vi "Power Output Compare and Coerce Stimulus.vi"(6 "Driver Ref (null)":T1, 8 "error in (no error)":errorcluster, 10 "Flat TestSetDef Params":string, 11 "PV Test Parameters":T2={"Stimulus"={"Frequency Type"=enum."Band Edges", "Frequency Ranges"=[], "TX 1 Frequency (MHz)"={"Min"=0.0, "Max"=0.0}, "TX 2 Frequency (MHz)"={"Min"=0.0, "Max"=0.0}, "RX Frequency (MHz)"={"Min"=0.0, "Max"=0.0}, "Pad Model Number"="", "Pad Serial Number"="", "Pad Values"=[]}, "Measurement"={"DUT Port"=enum."Port 1", "Direction"=0, "Frequency Step Size"=0}, "Display"={"Frequency"={"Min"=-1.0, "Max"=-1.0}, "Power"={"Min"=-1, "Max"=-1}}, "Limit"={"Min Power (dBm)"=44.0}, "Calibration"={"Calibrated?"=FALSE}} {"Measurement"."Frequency Step Size" items=["0.2", "0.4", "1.0", "2.0", "4.0"]; "Measurement"."Direction" items=["Reverse", "Forward", "Auxiliary"]}) -> (0 "error out":errorcluster, 3 "Corrected Test Params":T2={"Stimulus"={"Frequency Type"=enum."Band Edges", "Frequency Ranges"=[], "TX 1 Frequency (MHz)"={"Min"=0.0, "Max"=0.0}, "TX 2 Frequency (MHz)"={"Min"=0.0, "Max"=0.0}, "RX Frequency (MHz)"={"Min"=0.0, "Max"=0.0}, "Pad Model Number"="", "Pad Serial Number"="", "Pad Values"=[]}, "Measurement"={"DUT Port"=enum."Port 1", "Direction"=0, "Frequency Step Size"=0}, "Display"={"Frequency"={"Min"=-1.0, "Max"=-1.0}, "Power"={"Min"=-1, "Max"=-1}}, "Limit"={"Min Power (dBm)"=44.0}, "Calibration"={"Calibrated?"=FALSE}} {"Measurement"."Frequency Step Size" items=["0.2", "0.4", "1.0", "2.0", "4.0"]; "Measurement"."Direction" items=["Reverse", "Forward", "Auxiliary"]}, 4 "TestSetDef":T11={"General"={"ID"=0, "Model"="", "Dual Port?"=FALSE, "Options"="", "Options"={"E"=FALSE, "K"=FALSE, "H"=FALSE, "W"=FALSE, "F"=FALSE}, "Cal File"=path ""}, "Receiver"={"Fstart, MHz"=0.0, "Fstop MHz"=0.0, "Fstep MHz"=0.0, "IF, MHz"=0.0}, "RX Band"={"Fstart, MHz"=0.0, "Fstop MHz"=0.0}, "TX 1"={"Fstart, MHz"=0.0, "Fstop MHz"=0.0, "Pmax, dBm"=0.0, "Pstep, dB"=0.0}, "TX 2"={"Fstart, MHz"=0.0, "Fstop MHz"=0.0, "Pmax, dBm"=0.0, "Pstep, dB"=0.0}, "Low-side?"=TRUE})   [LabVIEW 2011]
uses:
  SI.LIB/PIM.LIB/HW IO/Test Set Definition.ctl
  TypeDefs/Power Output Test Parameters.ctl
  TypeDefs/Power Output Stimulus Parameters.ctl
  TypeDefs/Power Output Measurement Parameters.ctl
  SI.LIB/PIM.LIB/HW IO/DUTport.ctl
  SI.LIB/PIM.LIB/HW IO/MeasMode.ctl
  SI.LIB/PIM.LIB/HW IO/PIM Sweep Step Size.ctl
  TypeDefs/Power Output Display Parameters.ctl
  TypeDefs/Power Output Limit Parameters.ctl
  TypeDefs/Power Output Calibration State.ctl
  drivers/PIM/PIM Driver Ref.ctl
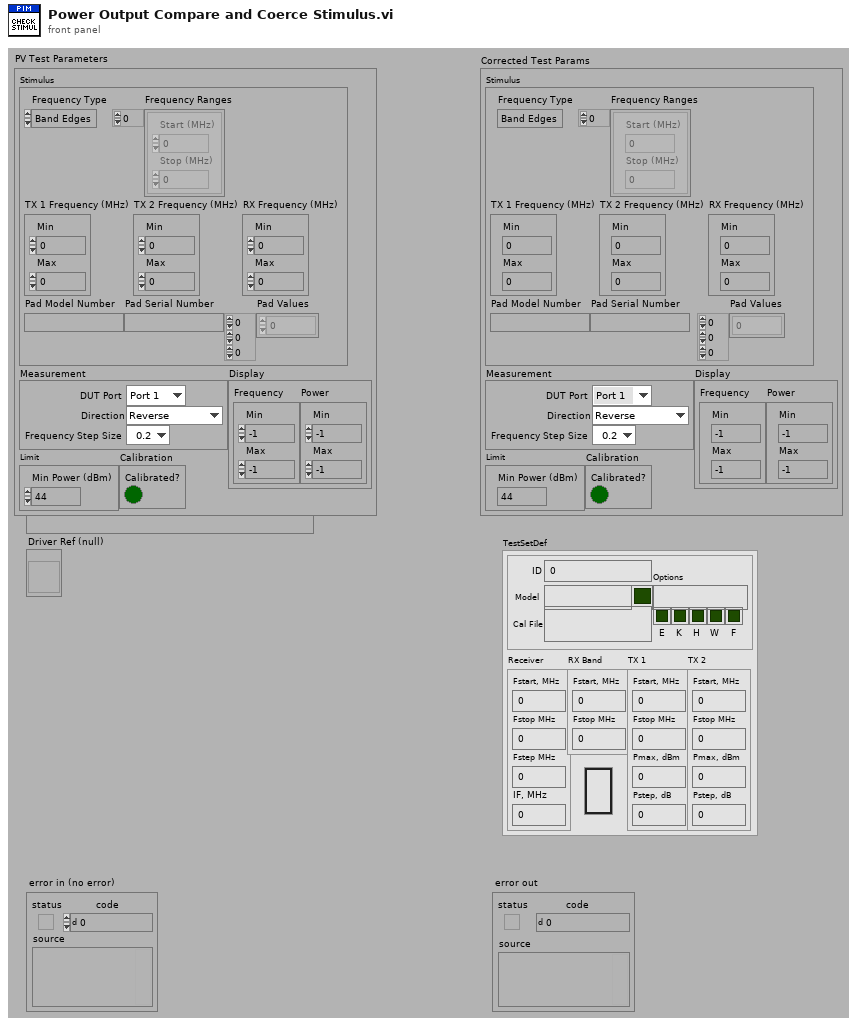
[diagram p1: front panel]
types:
  T1 = typedef "PIM Driver Ref.ctl" = refnum<vi>
  T2 = typedef "Power Output Test Parameters.ctl" = cluster{"Stimulus":T3, "Measurement":T4, "Display":T8, "Limit":T9, "Calibration":T10}
  T3 = typedef "Power Output Stimulus Parameters.ctl" = cluster{"Frequency Type":enum16{"Band Edges", "Custom"}, "Frequency Ranges":cluster{"Start (MHz)":dbl, "Stop (MHz)":dbl}[], "TX 1 Frequency (MHz)":cluster{"Min":dbl, "Max":dbl}, "TX 2 Frequency (MHz)":cluster{"Min":dbl, "Max":dbl}, "RX Frequency (MHz)":cluster{"Min":dbl, "Max":dbl}, "Pad Model Number":string, "Pad Serial Number":string, "Pad Values":dbl[][][]}
  T4 = typedef "Power Output Measurement Parameters.ctl" = cluster{"DUT Port":T5, "Direction":T6, "Frequency Step Size":T7}
  T5 = typedef "DUTport.ctl" = enum16{"Port 1", "Port 2"}
  T6 = typedef "MeasMode.ctl" = u16
  T7 = typedef "PIM Sweep Step Size.ctl" = u16
  T8 = typedef "Power Output Display Parameters.ctl" = cluster{"Frequency":cluster{"Min":dbl, "Max":dbl}, "Power":cluster{"Min":i32, "Max":i32}}
  T9 = typedef "Power Output Limit Parameters.ctl" = cluster{"Min Power (dBm)":dbl}
  T10 = typedef "Power Output Calibration State.ctl" = cluster{"Calibrated?":bool}
  T11 = typedef "Test Set Definition.ctl" = cluster{"General":cluster{"ID":u32, "Model":string, "Dual Port?":bool, "Options":string, "Options":cluster{"E":bool, "K":bool, "H":bool, "W":bool, "F":bool}, "Cal File":path}, "Receiver":cluster{"Fstart, MHz":dbl, "Fstop MHz":dbl, "Fstep MHz":dbl, "IF, MHz":dbl}, "RX Band":cluster{"Fstart, MHz":dbl, "Fstop MHz":dbl}, "TX 1":cluster{"Fstart, MHz":dbl, "Fstop MHz":dbl, "Pmax, dBm":dbl, "Pstep, dB":dbl}, "TX 2":cluster{"Fstart, MHz":dbl, "Fstop MHz":dbl, "Pmax, dBm":dbl, "Pstep, dB":dbl}, "Low-side?":bool}
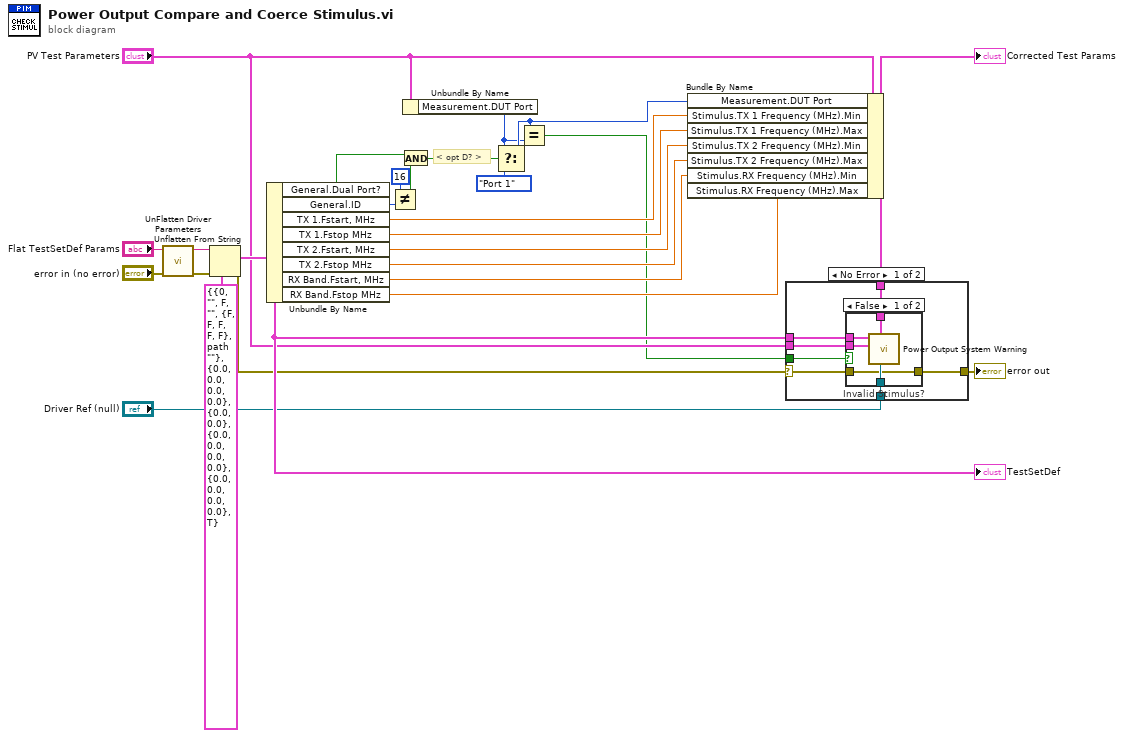
[diagram p0: block diagram]
diagram:
  # "< opt D? >"
  n1 = call "UnFlatten Driver Parameters.vi"("error in (no error)"="error in (no error)", "Flattened Driver Parameters with Version (\"\")"="Flat TestSetDef Params") -> ("error out"=w22:errorcluster, "Flat Driver Parameters"=w24:string)  [unwired: 4 out]
  n2 = Unflatten From String(type=T11 {"General"={"ID"=0, "Model"="", "Dual Port?"=FALSE, "Options"="", "Options"={"E"=FALSE, "K"=FALSE, "H"=FALSE, "W"=FALSE, "F"=FALSE}, "Cal File"=path ""}, "Receiver"={"Fstart, MHz"=0.0, "Fstop MHz"=0.0, "Fstep MHz"=0.0, "IF, MHz"=0.0}, "RX Band"={"Fstart, MHz"=0.0, "Fstop MHz"=0.0}, "TX 1"={"Fstart, MHz"=0.0, "Fstop MHz"=0.0, "Pmax, dBm"=0.0, "Pstep, dB"=0.0}, "TX 2"={"Fstart, MHz"=0.0, "Fstop MHz"=0.0, "Pmax, dBm"=0.0, "Pstep, dB"=0.0}, "Low-side?"=TRUE} ("Test Set Definition"), binary string=w24, error in (no error)=w22) -> (value=w21:T11, error out=w19:errorcluster)  [unwired: 3 out]
  "TestSetDef" <- w21
  n3 = Unbundle By Name(w21) -> ("General.Dual Port?"=w16:bool, "General.ID"=w12:u32, "TX 1.Fstart, MHz"=w8:dbl, "TX 1.Fstop MHz"=w7:dbl, "TX 2.Fstart, MHz"=w6:dbl, "TX 2.Fstop MHz"=w5:dbl, "RX Band.Fstart, MHz"=w4:dbl, "RX Band.Fstop MHz"=w3:dbl)
  n4 = Not Equal?(x=16 ("y"), y=w12) -> (x != y?=w17:bool)
  n5 = And(x=w16, y=w17) -> (x .and. y?=w14:bool)
  n6 = Unbundle By Name("PV Test Parameters") -> ("Measurement.DUT Port"=w10:T5)
  n7 = Select(t=w10, s=w14, f=DUTport."Port 1" ("Measure.DUT PORT")) -> (s? t:f=w11:T5)
  n8 = Equal?(x=w11, y=w10) -> (x = y?=w1:bool)
  n9 = Bundle By Name(cluster="PV Test Parameters", "Measurement.DUT Port"=w11, "Stimulus.TX 1 Frequency (MHz).Min"=w8, "Stimulus.TX 1 Frequency (MHz).Max"=w7, "Stimulus.TX 2 Frequency (MHz).Min"=w6, "Stimulus.TX 2 Frequency (MHz).Max"=w5, "Stimulus.RX Frequency (MHz).Min"=w4, "Stimulus.RX Frequency (MHz).Max"=w3) -> (w2:T2)
  "Corrected Test Params" <- w2
  n10 = case shown="No Error" w19 {
    selector: w19 -> [w29 w40]
    tunnel: w1 -> [w33 _]
    tunnel: w21 -> [w32 _]
    tunnel: [w31 w40] -> w20
    tunnel: "PV Test Parameters" -> [w30 _]
    tunnel: "Driver Ref (null)" -> [w28 _]
    tunnel: w2 -> [w27 _]
    frame No Error {
      n11 = case "Invalid Stimulus?" shown="False" w33 {
        tunnel: w32 -> [w38 _]
        tunnel: w30 -> [w37 _]
        tunnel: w29 -> [w35 w39]
        tunnel: [w35 w39] -> w31
        tunnel: w28 -> [w36 _]
        tunnel: w27 -> [w34 _]
        frame False {
          n12 = call "Power Output System Warning.vi"("Driver Ref (null)"=w36, "Coerced PV Test Parameters"=w34, "PV Test Parameters"=w37, "TestSetDef"=w38) -> ()  [unwired: 1 in, 7 out]
        }
        frame True {
        }
      }
    }
    frame Error {
      # "If we're in an error state, pass\nthe driver error through to the\nclient machine."
    }
  }
  "error out" <- w20
